vi "Save File Load Dialog Data.vi"(8 "error in (no error)":errorcluster, 10 "FileDialog":T2={"File"=path "", "Group"="", "Channel"="", "DataPlugin"="", "MissingTeeth"=0.0, "ErrState"="", "File Selected"=FALSE, "Data Selection Method"=enum."Manual", "Offset"=0, "Length"=0, "DataPlugins Info"=[], "Controls"=[], "File Ref"=refnum, "Groups"=[], "Channels"=[], "Groups Refs"=[], "Channel Refs"=[], "Cancelled"=FALSE, "Position reference"=enum."Crank angle", "FPGA memory size"=enum."32,768", "GroupRef"=refnum, "ChanRef"=refnum, "Data"=[], "ReverseData"=FALSE, "DispTwoRotations"=FALSE, "cycle range"=720}, 11 "Node Ptr":T1 format="%.0x") -> (0 "error out":errorcluster)   [LabVIEW 2015, in "Engine Simulation Toolkit System Explorer.lvlib"]
uses:
  Engine Simulation Toolkit System Explorer.lvlib
  File Load Dialog.ctl
  Data Replay Data Selection Method.ctl
  <vilib>/Platform/storage/utility/usiPluginInformation.ctl
  Position Reference.ctl
  FPGA Mem Size.ctl
  <vilib>/NI Veristand/Custom Device API/Custom Device Item Ref.ctl
  Shared/Properties.vi
  <vilib>/NI Veristand/Custom Device API/Set Item Property (Boolean).vi
  <vilib>/NI Veristand/Custom Device API/Set Item Property (Dependent File).vi
  <vilib>/NI Veristand/Custom Device API/Set Item Property (String).vi
  <vilib>/NI Veristand/Custom Device API/Set Item Property (Double).vi
  <vilib>/NI Veristand/Custom Device API/Set Item Property (I32).vi
  <vilib>/NI Veristand/Custom Device API/Set Item Property (U16).vi
  <vilib>/NI Veristand/Custom Device API/Custom Device API.lvlib
  Shared/Engine Simulation Toolkit Shared.lvlib
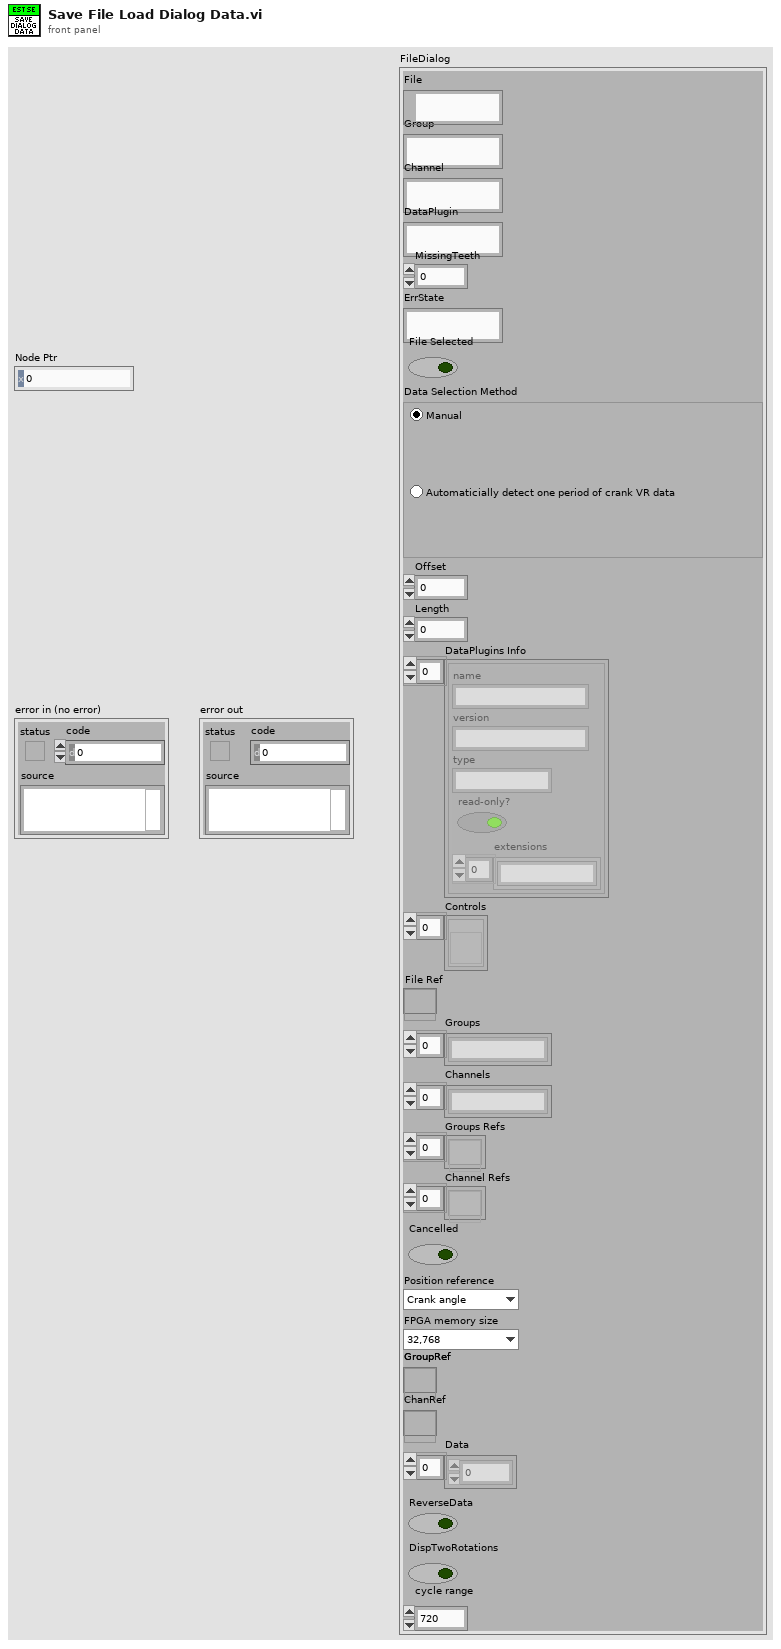
[diagram p1: front panel]
types:
  T1 = typedef "Custom Device API.lvlib/Custom Device Item Ref.ctl" = u64
  T2 = typedef "Engine Simulation Toolkit System Explorer.lvlib/File Load Dialog.ctl" = cluster{"File":path, "Group":string, "Channel":string, "DataPlugin":string, "MissingTeeth":dbl, "ErrState":string, "File Selected":bool, "Data Selection Method":T3, "Offset":i32, "Length":i32, "DataPlugins Info":T4[], "Controls":refnum<vi>[], "File Ref":refnum<k20>, "Groups":string[], "Channels":string[], "Groups Refs":refnum<k20>[], "Channel Refs":refnum<k20>[], "Cancelled":bool, "Position reference":T5, "FPGA memory size":T6, "GroupRef":refnum<k20>, "ChanRef":refnum<k20>, "Data":dbl[], "ReverseData":bool, "DispTwoRotations":bool, "cycle range":u16}
  T3 = typedef "Engine Simulation Toolkit System Explorer.lvlib/Data Replay Data Selection Method.ctl" = enum32{"Manual", "AutoVRCrank"}
  T4 = typedef "usiPluginInformation.ctl" = cluster{"name":string, "version":string, "type":string, "read-only?":bool, "extensions":string[]}
  T5 = typedef "Engine Simulation Toolkit System Explorer.lvlib/Position Reference.ctl" = enum16{"Crank angle", "Cycle angle"}
  T6 = typedef "Engine Simulation Toolkit System Explorer.lvlib/FPGA Mem Size.ctl" = enum16{"65,536", "32,768", "16,384", "8,192", "4,096", "2,048", "1,024"}
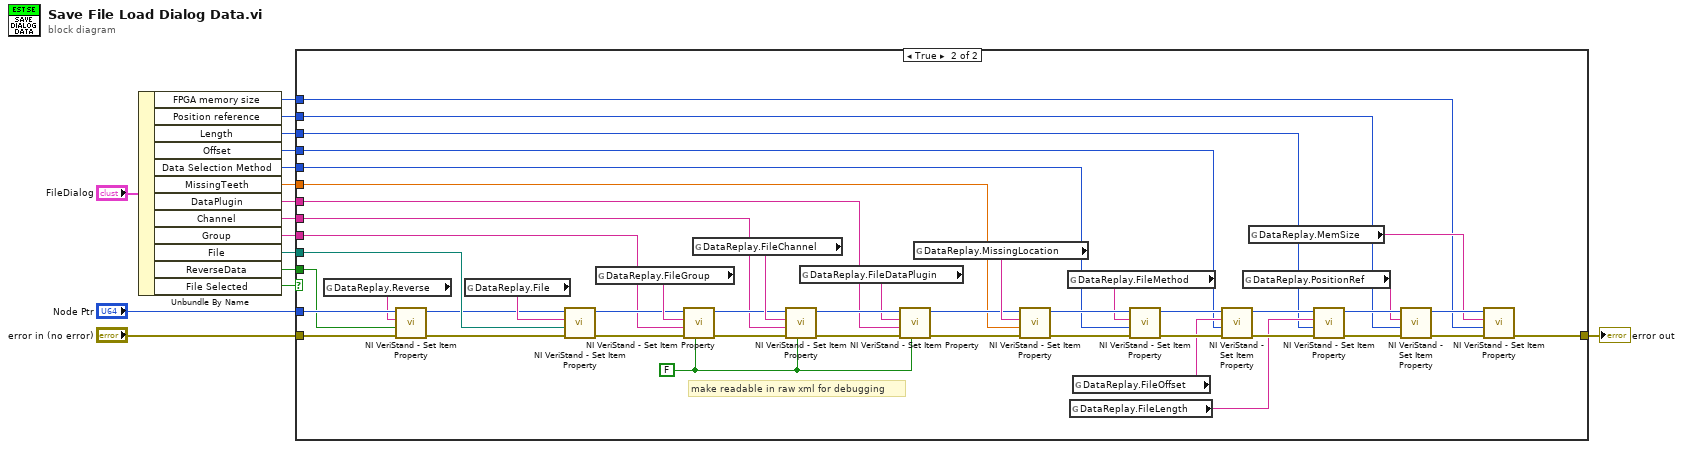
[diagram p0: block diagram]
diagram:
  n1 = Unbundle By Name("FileDialog") -> ("FPGA memory size"=w1:T6, "Position reference"=w2:T5, "Length"=w4:i32, "Offset"=w5:i32, "Data Selection Method"=w6:T3, "MissingTeeth"=w7:dbl, "DataPlugin"=w8:string, "Channel"=w9:string, "Group"=w10:string, "File"=w11:path, "ReverseData"=w3:bool, "File Selected"=w12:bool)
  n2 = case shown="True" w12 {
    tunnel: "Node Ptr" -> [_ w30]
    tunnel: "error in (no error)" -> [w17 w42]
    tunnel: [w17 w22] -> w16
    tunnel: w11 -> [_ w40]
    tunnel: w10 -> [_ w39]
    tunnel: w9 -> [_ w38]
    tunnel: w8 -> [_ w37]
    tunnel: w7 -> [_ w36]
    tunnel: w6 -> [_ w35]
    tunnel: w5 -> [_ w34]
    tunnel: w4 -> [_ w33]
    tunnel: w3 -> [_ w27]
    tunnel: w2 -> [_ w20]
    tunnel: w1 -> [_ w18]
    frame False {
    }
    frame True {
      w32 = FALSE ("Binary String (T)")
      # "make readable in raw xml for debugging"
      n3 = global read "Properties.vi" "DataReplay.Reverse"() -> (w28:string)
      n4 = call-poly <vilib>:"NI VeriStand - Set Item Property.vi"("error in (no error)"=w42, "Value"=w27, "Property Name"=w28, "Item Ref in"=w30) -> ("error out"=w31:errorcluster, "Item Ref out"=w29:T1)  [unwired: 5 in, 1 out]
      n5 = global read "Properties.vi" "DataReplay.File"() -> (w41:string)
      n6 = call-poly <vilib>:"NI VeriStand - Set Item Property.vi"("error in (no error)"=w31, "Path"=w40, "Property Name"=w41, "Item Ref in"=w29) -> ("error out"=w43:errorcluster, "Item Ref out"=w44:T1)  [unwired: 5 in, 1 out]
      n7 = global read "Properties.vi" "DataReplay.FileGroup"() -> (w63:string)
      n8 = call-poly <vilib>:"NI VeriStand - Set Item Property.vi"("Binary String (T)"=w32, "error in (no error)"=w43, "Value"=w39, "Property Name"=w63, "Item Ref in"=w44) -> ("error out"=w60:errorcluster, "Item Ref out"=w61:T1)  [unwired: 4 in, 1 out]
      n9 = global read "Properties.vi" "DataReplay.FileChannel"() -> (w62:string)
      n10 = call-poly <vilib>:"NI VeriStand - Set Item Property.vi"("Binary String (T)"=w32, "error in (no error)"=w60, "Value"=w38, "Property Name"=w62, "Item Ref in"=w61) -> ("error out"=w58:errorcluster, "Item Ref out"=w59:T1)  [unwired: 4 in, 1 out]
      n11 = global read "Properties.vi" "DataReplay.FileDataPlugin"() -> (w57:string)
      n12 = call-poly <vilib>:"NI VeriStand - Set Item Property.vi"("Binary String (T)"=w32, "error in (no error)"=w58, "Value"=w37, "Property Name"=w57, "Item Ref in"=w59) -> ("error out"=w54:errorcluster, "Item Ref out"=w55:T1)  [unwired: 4 in, 1 out]
      n13 = global read "Properties.vi" "DataReplay.MissingLocation"() -> (w56:string)
      n14 = call-poly <vilib>:"NI VeriStand - Set Item Property.vi"("error in (no error)"=w54, "Value"=w36, "Property Name"=w56, "Item Ref in"=w55) -> ("error out"=w52:errorcluster, "Item Ref out"=w53:T1)  [unwired: 5 in, 1 out]
      n15 = global read "Properties.vi" "DataReplay.FileMethod"() -> (w51:string)
      n16 = global read "Properties.vi" "DataReplay.FileLength"() -> (w45:string)
      n17 = global read "Properties.vi" "DataReplay.FileOffset"() -> (w46:string)
      n18 = call-poly <vilib>:"NI VeriStand - Set Item Property.vi"("error in (no error)"=w52, "Value"=w35, "Property Name"=w51, "Item Ref in"=w53) -> ("error out"=w49:errorcluster, "Item Ref out"=w50:T1)  [unwired: 5 in, 1 out]
      n19 = call-poly <vilib>:"NI VeriStand - Set Item Property.vi"("error in (no error)"=w49, "Value"=w34, "Property Name"=w46, "Item Ref in"=w50) -> ("error out"=w47:errorcluster, "Item Ref out"=w48:T1)  [unwired: 5 in, 1 out]
      n20 = global read "Properties.vi" "DataReplay.PositionRef"() -> (w21:string)
      n21 = global read "Properties.vi" "DataReplay.MemSize"() -> (w19:string)
      n22 = call-poly <vilib>:"NI VeriStand - Set Item Property.vi"("error in (no error)"=w47, "Value"=w33, "Property Name"=w45, "Item Ref in"=w48) -> ("error out"=w24:errorcluster, "Item Ref out"=w26:T1)  [unwired: 5 in, 1 out]
      n23 = call-poly <vilib>:"NI VeriStand - Set Item Property.vi"("error in (no error)"=w24, "Value"=w20, "Property Name"=w21, "Item Ref in"=w26) -> ("error out"=w23:errorcluster, "Item Ref out"=w25:T1)  [unwired: 5 in, 1 out]
      n24 = call-poly <vilib>:"NI VeriStand - Set Item Property.vi"("error in (no error)"=w23, "Value"=w18, "Property Name"=w19, "Item Ref in"=w25) -> ("error out"=w22:errorcluster)  [unwired: 5 in, 2 out]
    }
  }
  "error out" <- w16
